vi "A170316-11.vi"() -> ()   [LabVIEW 2020]
panel:
  in  "电机安装LED":refnum<vi>[](array[refnum])
  in  "控制器支架LED":refnum<vi>[](array[refnum])
  in  "安装支架LED":refnum<vi>[](array[refnum])
  in  "顶板类型":enum32{"Radio Selection 1", "Radio Selection 2"}(radio)
  in  "啮合间隙判定参数":cluster{"最大值":string, "最小值":string}
  in  "啮合曲线":refnum<vi>
  in  "磨合次数":i32
  in  "磨合曲线":refnum<vi>
  in  "空载曲线":refnum<vi>
  in  "空载逆向判定参数":T1
  in  "空载正向判定参数":T1
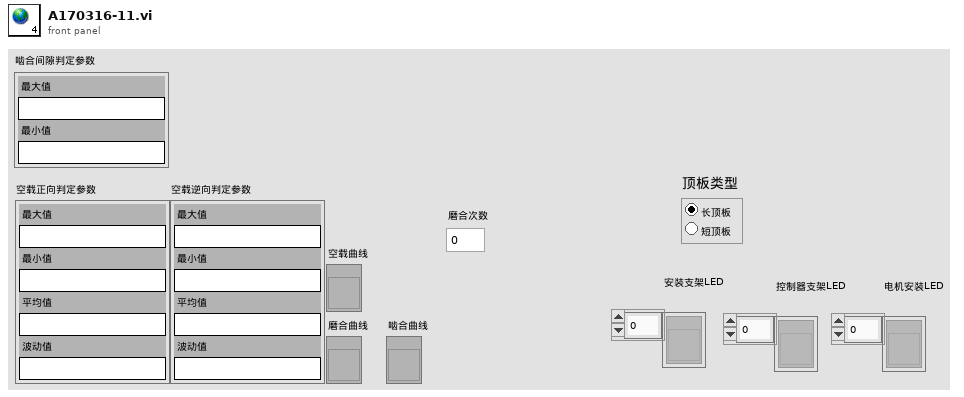
[diagram p1: front panel]
types:
  T1 = cluster{"最大值":string, "最小值":string, "平均值":string, "波动值":string}
diagram:
